vi "Convert xyz hex strings into decimal coordinates.vi"(11 "read string":string="@\u0006\u0000\u0000€\f\u0000\u0000À\u0012\u0000\u0000\r") -> (0 "Zcoordinate (not rounded)":dbl format="%.4f", 1 "Zcoordinate":i32, 2 "Ycoordinate":i32, 3 "Xcoordinate":i32, 4 "Ycoordinate (not rounded)":dbl format="%.4f", 6 "Xcoordinate (not rounded)":dbl format="%.4f")   [LabVIEW 2010]
panel:
  out "Zcoordinate":string
  out "Ycoordinate":string
  out "Xcoordinate":string
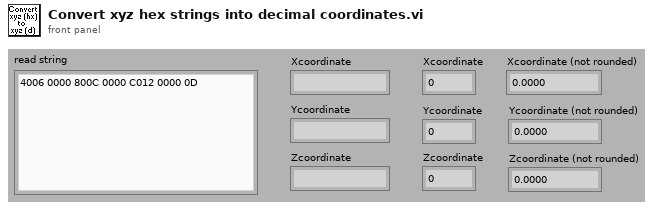
[diagram p1: front panel]
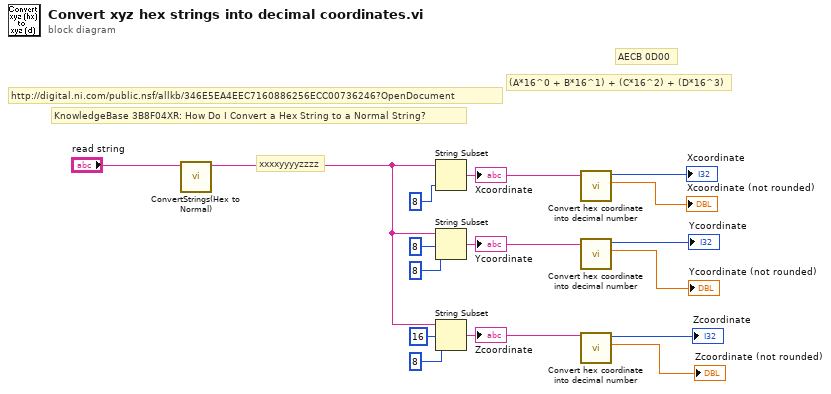
[diagram p0: block diagram]
diagram:
  # "xxxxyyyyzzzz"
  # "(A*16^0 + B*16^1) + (C*16^2) + (D*16^3)"
  # "AECB 0D00"
  # "http://digital.ni.com/public.nsf/allkb/346E5EA4EEC7160886256ECC00736246?OpenDocument"
  # "KnowledgeBase 3B8F04XR: How Do I Convert a Hex String to a Normal String?"
  n1 = call "ConvertStrings(Hex to Normal).vi"("Hex String"="read string") -> ("Normal String"=w12:string)  [unwired: 10 out]
  n2 = String Subset(string=w12, length (rest)=8 ("length (rest)")) -> (substring=w9:string)  [unwired: 1 out]
  "Xcoordinate" <- w9
  n3 = String Subset(string=w12, offset (0)=8, length (rest)=8 ("length (rest)")) -> (substring=w8:string)
  "Ycoordinate" <- w8
  n4 = String Subset(string=w12, offset (0)=16, length (rest)=8 ("length (rest)")) -> (substring=w7:string)
  "Zcoordinate" <- w7
  n5 = call "Convert hex coordinate into decimal number.vi"("Coordinate"=w9) -> ("Decimal number (not rounded)"=→"Xcoordinate (not rounded)":dbl, "Decimal number (rounded)"=→"Xcoordinate":i32)  [unwired: 9 out]
  n6 = call "Convert hex coordinate into decimal number.vi"("Coordinate"=w8) -> ("Decimal number (not rounded)"=→"Ycoordinate (not rounded)":dbl, "Decimal number (rounded)"=→"Ycoordinate":i32)  [unwired: 9 out]
  n7 = call "Convert hex coordinate into decimal number.vi"("Coordinate"=w7) -> ("Decimal number (not rounded)"=→"Zcoordinate (not rounded)":dbl, "Decimal number (rounded)"=→"Zcoordinate":i32)  [unwired: 9 out]
